vi "Create Last Temperature Entry.vi"(8 "error in":errorcluster, 10 "Channel":string, 11 "Thermometer DAQmx RTD Cont CFG in":refnum<class "Thermometer DAQmx RTD Cont CFG.lvclass">) -> (0 "error out":errorcluster, 3 "Thermometer DAQmx RTD Cont CFG out":refnum<class "Thermometer DAQmx RTD Cont CFG.lvclass">)   [LabVIEW 2023, in "Thermometer DAQmx RTD Cont CFG.lvclass"]
uses:
  Thermometer DAQmx RTD Cont CFG.lvclass
  Thermometer DAQmx RTD Cont CFG.lvclass/Thermometer DAQmx RTD Cont CFG.ctl
  <vilib>/Utility/miscctls.llb/LVMapReplaceAction.ctl
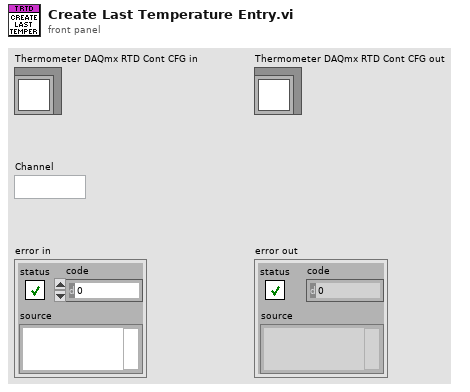
[diagram p1: front panel]
types:
  T1 = typedef "LVMapReplaceAction.ctl" = enum32{"Modify Entry only if found", "Add or Modify Entry", "Delete Entry"}
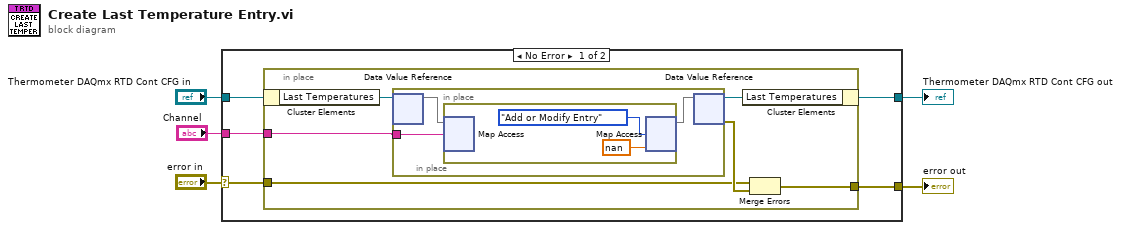
[diagram p0: block diagram]
diagram:
  n1 = case shown="No Error" "error in" {
    selector: "error in" -> [w8 w23]
    tunnel: [w7 w23] -> w4
    tunnel: [w6 w22] -> w2
    tunnel: "Thermometer DAQmx RTD Cont CFG in" -> [w10 w22]
    tunnel: "Channel" -> [w9 _]
    frame No Error {
      n2 = in-place {
        in-place-border: w9 -> [w15]
        in-place-border: w8 -> [w13]
        in-place-border: [w12] -> w7
        n3 = in-place-cluster #1(w10) -> ("Last Temperatures"=w16:refnum<data-value>)
        n4 = in-place {
          in-place-border: w15 -> [w18]
          n5 = in-place-dvr #2(w16) -> (w19:map{string, dbl})  [unwired: 1 out]
          n6 = in-place {
            n7 = in-place-map #3(w19, w18) -> ()  [unwired: 1 in, 2 out]
            n8 = in-place-map #3(nan, LVMapReplaceAction."Add or Modify Entry" ("action")) -> (w17:map{string, dbl})  [unwired: 2 out]
          }
          n9 = in-place-dvr #2(w17) -> (w11:refnum<data-value>, w14:errorcluster)
        }
        n10 = in-place-cluster #1("Last Temperatures"=w11) -> (w6:refnum<class "Thermometer DAQmx RTD Cont CFG.lvclass">)
        n11 = Merge Errors(w13, w14) -> (w12:errorcluster)
      }
    }
    frame Error {
    }
  }
  "error out" <- w4
  "Thermometer DAQmx RTD Cont CFG out" <- w2
